vi "_test.vi"() -> ()   [LabVIEW 2020]
uses:
  <instrlib>/Agilent B2900 Series/Agilent B2900 Series.lvlib
panel:
  out "Measurement Result":dbl
  out "COMMAND":string
  in  "Measure":enum16{"Current", "Voltage", "Resistance"}(ring)
  in  "Source Voltage(V)":dbl
  in  "Channel":u32(ring) items=["", "1", "2"]
  out "Measurement":dbl
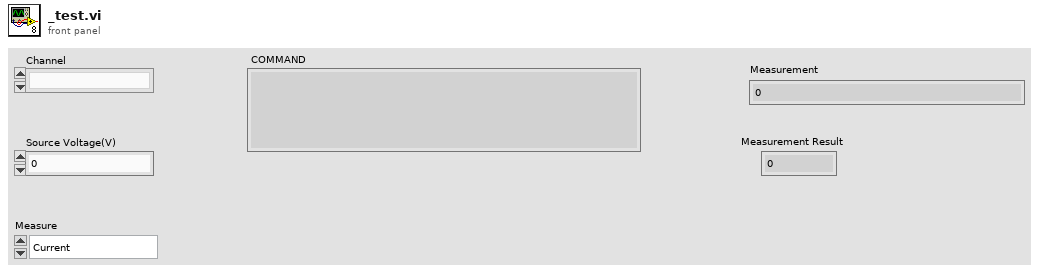
[diagram p1: front panel]
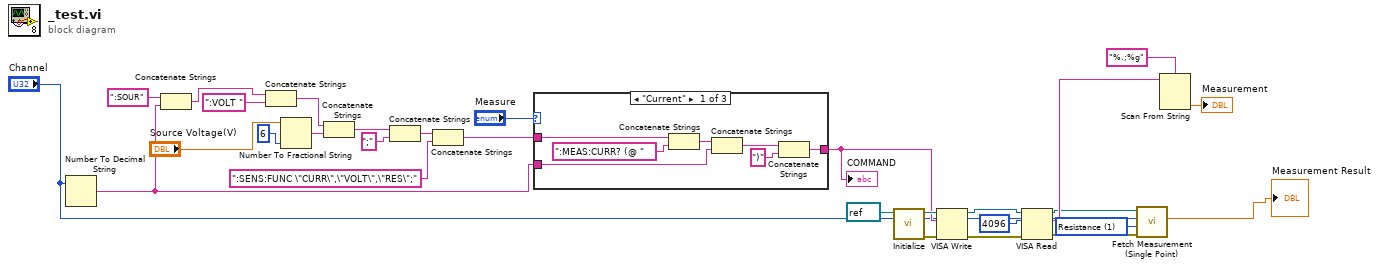
[diagram p0: block diagram]
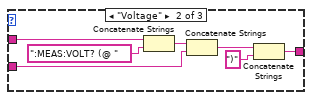
[diagram p2: hidden frame]
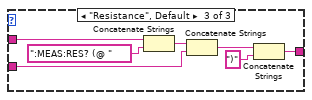
[diagram p3: hidden frame]
diagram:
  w2 = 1 items=["Current", "Resistance", "Source Output Setting", "Status", "Time", "Voltage"] ("Data Mode (5: Voltage)")
  n1 = Number To Decimal String(number="Channel") -> (decimal integer string=w8:string)  [unwired: 1 in]
  n2 = Concatenate Strings(":SOUR", w8) -> (w20:string)
  n3 = Concatenate Strings(w20, ":VOLT ") -> (w18:string)
  n4 = Number To Fractional String(number="Source Voltage(V)", precision (6)=i16 6) -> (F-format string=w13:string)  [unwired: 2 in]
  n5 = Concatenate Strings(w18, w13) -> (w17:string)
  n6 = Concatenate Strings(w17, ";" ("string")) -> (w12:string)
  n7 = Concatenate Strings(w12, ":SENS:FUNC \"CURR\",\"VOLT\",\"RES\";") -> (w9:string)
  n8 = case shown="\"Current\"" "Measure" {
    tunnel: w9 -> [w32 w43 w46]
    tunnel: w8 -> [w31 w40 w45]
    tunnel: [w30 w37 w44] -> w7
    frame "Current" {
      n9 = Concatenate Strings(w32, ":MEAS:CURR? (@ " ("string")) -> (w35:string)
      n10 = Concatenate Strings(w35, w31) -> (w34:string)
      n11 = Concatenate Strings(w34, ")" ("string")) -> (w30:string)
    }
    frame "Voltage" {
      n12 = Concatenate Strings(w43, ":MEAS:VOLT? (@ " ("string")) -> (w41:string)
      n13 = Concatenate Strings(w41, w40) -> (w39:string)
      n14 = Concatenate Strings(w39, ")" ("string")) -> (w37:string)
    }
    frame "Resistance", Default {
      n15 = Concatenate Strings(w46, ":MEAS:RES? (@ " ("string")) -> (w49:string)
      n16 = Concatenate Strings(w49, w45) -> (w48:string)
      n17 = Concatenate Strings(w48, ")" ("string")) -> (w44:string)
    }
  }
  "COMMAND" <- w7
  n18 = call <instrlib>:"Initialize.vi"("VISA resource name"=refnum<visa-resource-name> "USB0::0x0957::0x8E18::MY51140695::INSTR") -> ("error out"=w6:errorcluster, "VISA resource name out"=w25:refnum<visa-resource-name>)  [unwired: 9 in]
  n19 = VISA Write(VISA resource name=w25, write buffer=w7, error in (no error)=w6) -> (VISA resource name out=w28:refnum<visa-resource-name>, error out=w27:errorcluster)  [unwired: 1 out]
  n20 = VISA Read(VISA resource name=w28, byte count=u32 4096, error in (no error)=w27) -> (VISA resource name out=w5:refnum<visa-resource-name>, read buffer=w22:string, error out=w4:errorcluster)  [unwired: 1 out]
  n21 = call <instrlib>:"Fetch Measurement (Single Point).vi"("error in (no error)"=w4, "Data Mode (5: Voltage)"=w2, "Channel (0: Channel 1)"="Channel", "VISA resource name"=w5) -> ("Measurement"=→"Measurement Result":dbl)  [unwired: 5 in, 2 out]
  n22 = Scan From String(format string="%.;%g", input string=w22) -> (output 1=→"Measurement":dbl)  [unwired: 3 in, 3 out]
